vi "send.folder.volume.map.vi"(8 "error in (no error)":errorcluster, 9 "vol_map notifier":refnum<notifier>, 11 "manager_daemon in":refnum<class "manager_daemon.lvclass">) -> (0 "error out":errorcluster, 3 "manager_daemon out":refnum<class "manager_daemon.lvclass">)   [LabVIEW 2024, in "manager_daemon.lvclass"]
uses:
  manager_daemon.lvclass
  manager_daemon.lvclass/manager_daemon.ctl
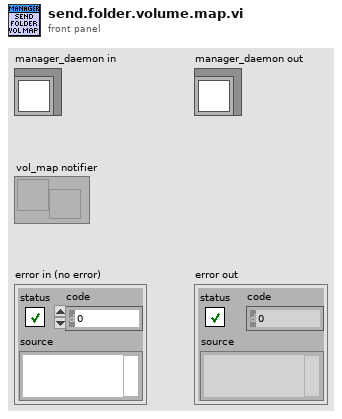
[diagram p1: front panel]
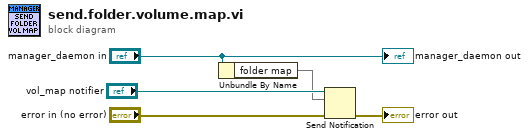
[diagram p0: block diagram]
diagram:
  n1 = Unbundle By Name("manager_daemon in") -> ("folder map"=w1:map{i32, map{string, i32}})
  n2 = Send Notification(notification=w1, notifier="vol_map notifier", error in (no error)="error in (no error)") -> (error out=→"error out":errorcluster)  [unwired: 1 out]
  "manager_daemon out" <- "manager_daemon in"
